vi "Servo MSMT TDSCDMA Set RF WFM Parameters.vi"(8 "error in (no error)":errorcluster, 10 "Step In":refnum<k7>, 11 "Servo MSMT in":refnum<class "Servo MSMT.lvclass">) -> (0 "error out":errorcluster, 2 "Step Out":refnum<k7>, 3 "Servo MSMT out":refnum<class "Servo MSMT.lvclass">)   [LabVIEW 2018, in "Servo MSMT.lvlib" / "Servo MSMT.lvclass"]
uses:
  Servo MSMT.lvclass
  C:/Sequence Automation/Plugins/Measurement Interface.lvlibp/Measurement Interface.lvclass
  Plugins/Measurement Interface.lvlibp/Private Methods/Measurement Parameters/Read Measurement Parameters.vi
  Plugins/String Database.lvlibp/String Database.lvclass
  Plugins/TestStand API Tools (TSAT).lvlibp/Step Actions/TSAT Step Actions.lvlib
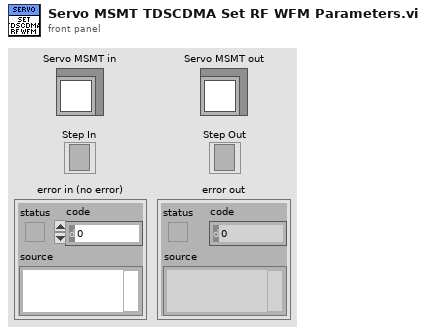
[diagram p1: front panel]
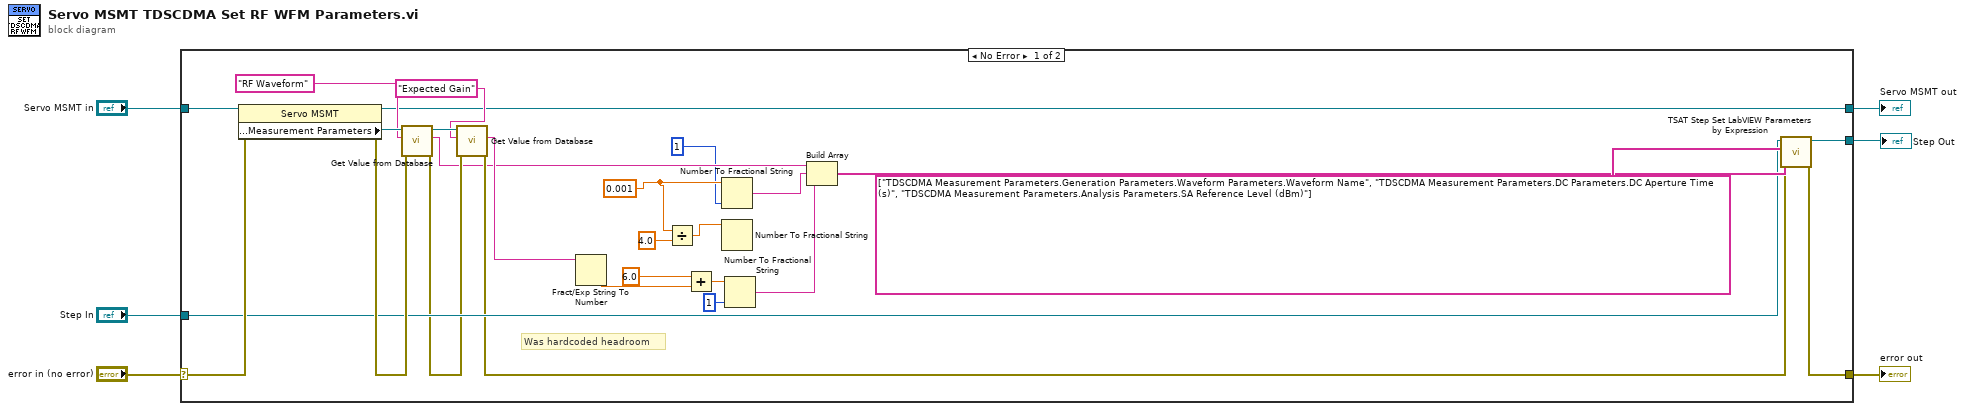
[diagram p0: block diagram]
diagram:
  n1 = case shown="No Error" "error in (no error)" {
    selector: "error in (no error)" -> [w33 w36]
    tunnel: [w30 w36] -> w5
    tunnel: [w11 w35] -> w3
    tunnel: "Servo MSMT in" -> [w29 w35]
    tunnel: [w22 w34] -> w2
    tunnel: "Step In" -> [w21 w34]
    frame No Error {
      w8 = 0.001 ("number")
      # "Was hardcoded headroom"
      n2 = property class="Servo MSMT"(reference=w29, error in=w33) -> (reference out=w11:refnum<class "Servo MSMT.lvclass">, error out=w27:errorcluster, "Protected Methods:Measurement Parameters"=w28:refnum<class "String Database.lvclass">)
      n3 = call "Get Value from Database.vi"("error in (no error)"=w27, "Entry Name"="RF Waveform", "Message in"=w28) -> ("error out"=w19:errorcluster, "Entry Value"=w9:string, "Message out"=w20:refnum<class "String Database.lvclass">)  [unwired: 5 in, 1 out]
      n4 = call "Get Value from Database.vi"("error in (no error)"=w19, "Entry Name"="Expected Gain", "Message in"=w20) -> ("error out"=w18:errorcluster, "Entry Value"=w16:string)  [unwired: 5 in, 2 out]
      n5 = Fract/Exp String To Number(string=w16) -> (number=w15:dbl)  [unwired: 3 in, 1 out]
      n6 = Divide(x=w8, y=4.0) -> (x/y=w31:dbl)
      n7 = Add(x=6.0 ("number"), y=w15) -> (x+y=w14:dbl)
      n8 = Number To Fractional String(number=w8, precision (6)=i16 1) -> (F-format string=w25:string)  [unwired: 2 in]
      n9 = Number To Fractional String(number=w31) -> ()  [unwired: 3 in, 1 out]
      n10 = Number To Fractional String(number=w14, precision (6)=i16 1) -> (F-format string=w13:string)  [unwired: 2 in]
      n11 = Build Array(w9, w25, w13) -> (w23:string[])
      n12 = call "TSAT Step Set LabVIEW Parameters by Expression.vi"("Error In"=w18, "Value Expressions"=w23, "Parameters to Set"=string[] ["TDSCDMA Measurement Parameters.Generation Parameters.Waveform Parameters.Waveform Name", "TDSCDMA Measurement Parameters.DC Parameters.DC Aperture Time (s)", "TDSCDMA Measurement Parameters.Analysis Parameters.SA Reference Level (dBm)"], "Step In"=w21) -> ("Error Out"=w30:errorcluster, "Step Out"=w22:refnum<k7>)  [unwired: 6 in]
    }
    frame Error {
    }
  }
  "error out" <- w5
  "Servo MSMT out" <- w3
  "Step Out" <- w2
